vi "Receive DS Packet.vi"(0 "Recv Socket":refnum<k16>, 1 "Log User Data":bool) -> (7 "Camera IP Address":string="10.0.0.2", 9 "Camera IP Address 2":string, 10 "New Dashboard Data":bool, 11 "Low Priority User Data":string, 12 "Battery":sgl, 13 "High Priority User Data":string, 14 "Error Strings":string, 15 "Driver Station":T1, 17 "Robot IP Address":string="10.0.0.2", 18 "Status":T3, 19 "Error":T2)   [LabVIEW 2012]
uses:
  DStoPCPacketTypeDef.ctl
panel:
  out "CRC":string
  out "Team ID":u16
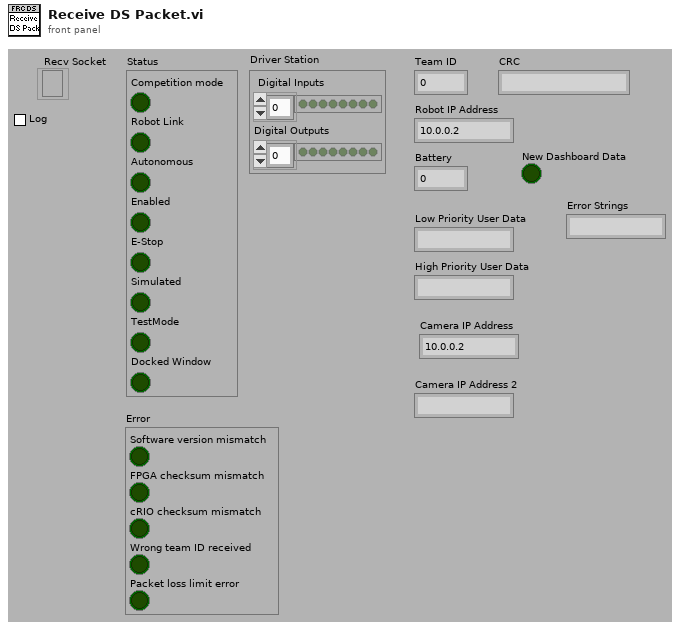
[diagram p1: front panel]
types:
  T1 = cluster{"Digital Inputs":bool[], "Digital Outputs":bool[]}
  T2 = cluster{"Software version mismatch":bool, "FPGA checksum mismatch":bool, "cRIO checksum mismatch":bool, "Wrong team ID received":bool, "Packet loss limit error":bool}
  T3 = cluster{"Competition mode":bool, "Robot Link":bool, "Autonomous":bool, "Enabled":bool, "E-Stop":bool, "Simulated":bool, "TestMode":bool, "Docked Window":bool}
  T4 = typedef "DStoPCPacketTypeDef.ctl" = cluster{"Packet Index":u16, "Digital Inputs":u8, "Digital Out":u8, "Battery":u16, "Status":u8, "Error":u8, "Team ID":u16, "VersionMonth1":u8, "VersionMonth2":u8, "VersionDay1":u8, "VersionDay2":u8, "VersionYear1":u8, "VersionYear2":u8, "Revision1":u8, "Revision2":u8, "Robot IP":u32, "UnusedBuffer 2":u8, "ExtraModeFlags":u8, "Reply Packet #":u16}
  T5 = cluster{"Boolean array":bool[], "Boolean array":bool[]}
  T6 = cluster{"Boolean array[0]":bool, "Boolean array[1]":bool, "Boolean array[2]":bool, "Boolean array[3]":bool, "Boolean array[4]":bool, "Boolean array[5]":bool, "Boolean array[6]":bool, "Boolean array[7]":bool}
  T7 = cluster{"Boolean array[0]":bool, "Boolean array[1]":bool, "Boolean array[4]":bool, "Boolean array[5]":bool, bool, bool, bool, bool}
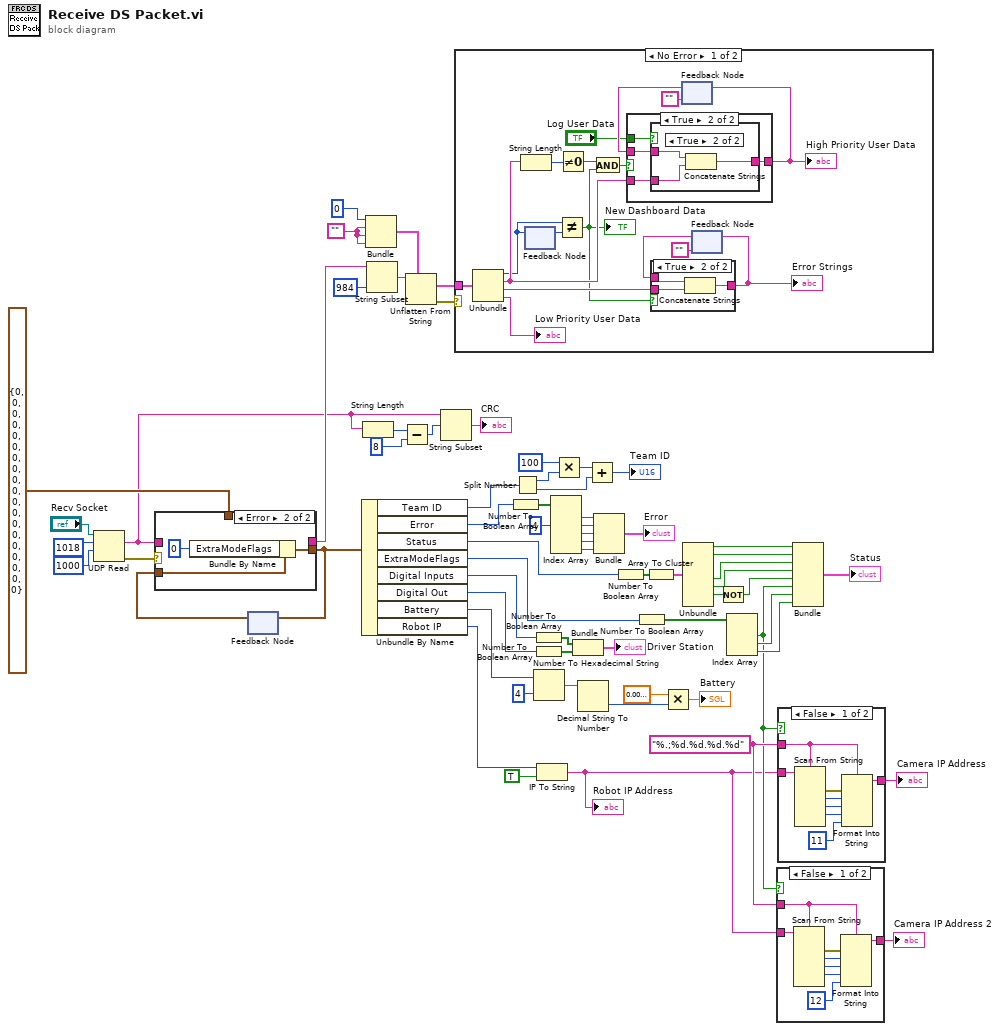
[diagram p0: block diagram]
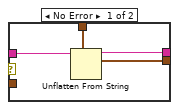
[diagram p3: hidden frame]
diagram:
  w4 = "%.;%d.%d.%d.%d" ("format string")
  w17 = ""
  n1 = UDP Read(connection ID="Recv Socket", max size (548)=1018 ("bytes to read"), timeout ms (25000)=1000) -> (data out=w6:string, error out=w10:errorcluster)  [unwired: 1 in, 3 out]
  n2 = feedback #1() -> (w9:T4)  [unwired: 1 in]
  n3 = case shown="Error" w10 {
    tunnel: w6 -> [w71 _]
    tunnel: w9 -> [_ w73]
    tunnel: [w70 w74] -> w5
    tunnel: T4 {"Packet Index"=0, "Digital Inputs"=0, "Digital Out"=0, "Battery"=0, "Status"=0, "Error"=0, "Team ID"=0, "VersionMonth1"=0, "VersionMonth2"=0, "VersionDay1"=0, "VersionDay2"=0, "VersionYear1"=0, "VersionYear2"=0, "Revision1"=0, "Revision2"=0, "Robot IP"=0, "UnusedBuffer 2"=0, "ExtraModeFlags"=0, "Reply Packet #"=0} ("Cluster") -> [w69 _]
    tunnel: [w68 _] -> w7
    frame No Error {
      n4 = Unflatten From String(type=w69, binary string=w71) -> (rest of the binary string=w68:string, value=w70:T4)  [unwired: 1 in, 3 out]
    }
    frame Error {
      n5 = Bundle By Name(cluster=w73, "ExtraModeFlags"=u8 0) -> (w74:T4)
    }
  }
  n6 = feedback-in #1(w5) -> ()
  n7 = Unbundle By Name(w5) -> ("Team ID"=w51:u16, "Error"=w59:u8, "Status"=w67:u8, "ExtraModeFlags"=w16:u8, "Digital Inputs"=w25:u8, "Digital Out"=w24:u8, "Battery"=w43:u16, "Robot IP"=w11:u32)
  n8 = String Length(string=w6) -> (length=w48:i32)
  n9 = Bundle(u8 0, w17, w17, w17) -> (w21:cluster{u8, string, string, string})  [unwired: 1 out]
  n10 = String Subset(string=w7, length (rest)=984 ("length (rest)")) -> (substring=w26:string)  [unwired: 1 out]
  n11 = Subtract(x=w48, y=8) -> (x-y=w46:i32)
  n12 = Unflatten From String(type=w21, binary string=w26) -> (value=w19:cluster{u8, string, string, string}, error out=w18:errorcluster)  [unwired: 1 in, 3 out]
  n13 = String Subset(string=w6, offset (0)=w46) -> (substring=→"CRC":string)  [unwired: 1 out]
  n14 = case shown="No Error" w18 {
    tunnel: w19 -> [w88 _]
    frame No Error {
      n15 = Unbundle(w88) -> (w79:u8, w80:string, w86:string, →"Low Priority User Data":string)
      n16 = String Length(string=w80) -> (length=w81:i32)
      n17 = feedback-in #2(w79) -> ()
      n18 = feedback #2() -> (w78:u8)  [unwired: 1 out]
      n19 = Not Equal?(x=w79, y=w78) -> (x != y?=w77:bool)
      "New Dashboard Data" <- w77
      n20 = Not Equal To 0?(x=w81) -> (x != 0?=w82:bool)
      n21 = And(x=w82, y=w77) -> (x .and. y?=w83:bool)
      n22 = feedback #3("") -> (w89:string)
      n23 = case shown="True" w83 {
        tunnel: w80 -> [_ w100]
        tunnel: [w96 w99] -> w75
        tunnel: w89 -> [w96 w98]
        tunnel: "Log User Data" -> [_ w97]
        frame False {
        }
        frame True {
          n24 = case shown="True" w97 {
            tunnel: w100 -> [w101 w104]
            tunnel: [w101 w103] -> w99
            tunnel: w98 -> [_ w102]
            frame False {
            }
            frame True {
              n25 = Concatenate Strings(w102, w104) -> (w103:string)
            }
          }
        }
      }
      "High Priority User Data" <- w75
      n26 = feedback-in #3(w75) -> ()
      n27 = feedback #4("") -> (w91:string)
      n28 = case shown="True" w77 {
        tunnel: [w92 w95] -> w76
        tunnel: w91 -> [w92 w94]
        tunnel: w86 -> [_ w93]
        frame False {
        }
        frame True {
          n29 = Concatenate Strings(w94, w93) -> (w95:string)
        }
      }
      "Error Strings" <- w76
      n30 = feedback-in #4(w76) -> ()
    }
    frame Error {
    }
  }
  n31 = Number To Boolean Array(number=w59) -> (Boolean array=w33:bool[])
  n32 = Split Number(x=w51) -> (hi(x)=w56:u8, lo(x)=w53:u8)
  n33 = Number To Boolean Array(number=w25) -> (Boolean array=w22:bool[])
  n34 = Number To Boolean Array(number=w24) -> (Boolean array=w23:bool[])
  n35 = Number To Hexadecimal String(1:i16 4 ("width (-)"), 2:w43) -> (0:w42:string)
  n36 = IP To String(1:TRUE ("dot notation? (F)"), 2:w11) -> (0:w2:string)
  "Robot IP Address" <- w2
  n37 = Index Array(array=w33, index #2=4 ("index")) -> (element #1=w27:bool, element #2=w28:bool, element #3=w29:bool, element #4=w30:bool, element #5=w31:bool)  [unwired: 4 in]
  n38 = Multiply(x=u16 100, y=w56) -> (x*y=w54:u16)
  n39 = Bundle("Boolean array"=w22, "Boolean array"=w23) -> (→"Driver Station":T5)  [unwired: 1 out]
  n40 = Decimal String To Number(string=w42) -> (number=w40:i32)  [unwired: 3 out]
  n41 = Add(x=w54, y=w53) -> (x+y=→"Team ID":u16)
  n42 = Bundle(w27, w28, w29, w30, w31) -> (→"Error":cluster{bool, bool, bool, bool, bool})  [unwired: 1 out]
  n43 = Number To Boolean Array(number=w67) -> (Boolean array=w66:bool[])
  n44 = Number To Boolean Array(number=w16) -> (Boolean array=w15:bool[])
  n45 = Array To Cluster(array=w66) -> (cluster=w64:T6)
  n46 = Multiply(x=sgl 0.01, y=w40) -> (x*y=→"Battery":sgl)
  n47 = Unbundle(w64) -> ("Boolean array[0]"=w63:bool, "Boolean array[1]"=w62:bool, "Boolean array[4]"=w61:bool, "Boolean array[5]"=w60:bool, "Boolean array[6]"=w58:bool)  [unwired: 3 out]
  n48 = Not(x=w58) -> (.not. x?=w57:bool)
  n49 = Index Array(array=w15) -> (element #1=w3:bool, element #2=w14:bool, element #3=w13:bool)  [unwired: 3 in]
  n50 = case shown="False" w3 {
    tunnel: [w107 w113] -> w1
    tunnel: w2 -> [w106 w113]
    tunnel: w4 -> [w105 _]
    frame False {
      n51 = Scan From String(format string=w105, input string=w106) -> (error out=w109:errorcluster, output 1=w110:i32, output 2=w111:i32, output 3=w112:i32)  [unwired: 2 in, 7 out]
      n52 = Format Into String(format string=w105, error in=w109, w110, w111, w112, 12 ("IP Suffix:")) -> (resulting string=w107:string)  [unwired: 1 in, 1 out]
    }
    frame True {
    }
  }
  "Camera IP Address 2" <- w1
  n53 = case shown="False" w3 {
    tunnel: [w116 w122] -> w12
    tunnel: w2 -> [w115 w122]
    tunnel: w4 -> [w114 _]
    frame False {
      n54 = Scan From String(format string=w114, input string=w115) -> (error out=w118:errorcluster, output 1=w119:i32, output 2=w120:i32, output 3=w121:i32)  [unwired: 2 in, 7 out]
      n55 = Format Into String(format string=w114, error in=w118, w119, w120, w121, 11 ("IP Suffix:")) -> (resulting string=w116:string)  [unwired: 1 in, 1 out]
    }
    frame True {
    }
  }
  "Camera IP Address" <- w12
  n56 = Bundle("Boolean array[0]"=w63, "Boolean array[1]"=w62, "Boolean array[4]"=w61, "Boolean array[5]"=w60, w57, w3, w14, w13) -> (→"Status":T7)  [unwired: 1 out]
